vi "MuxReset.vi"(8 "error in (no error)":errorcluster, 11 "Pickering in":refnum<class "Pickering.lvclass">) -> (0 "error out":errorcluster, 3 "Pickering out":refnum<class "Pickering.lvclass">)   [LabVIEW 2013, in "Pickering.lvclass"]
uses:
  Pickering.lvclass
  PickeringMUX_CommandsGlobal.vi
  InstrControl.lvclass
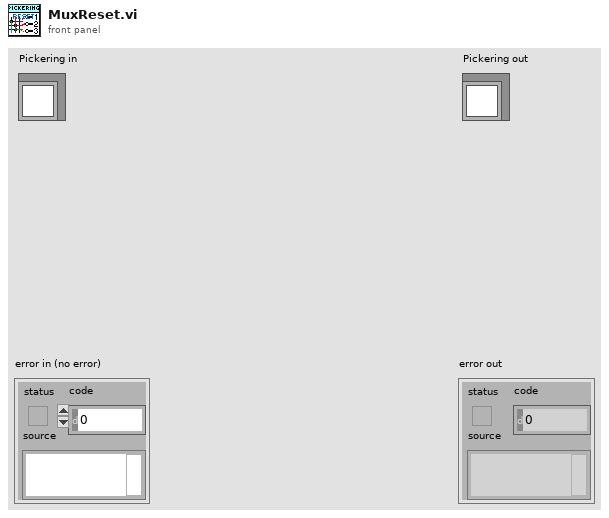
[diagram p1: front panel]
types:
  T1 = cluster{"Mux1 address":string, "Mux2 address":string, "Instrument name":string, "Instrument type":u16, "Command \"MUX Reset\"":string, "Command \"Select MUX Channel\"":string}
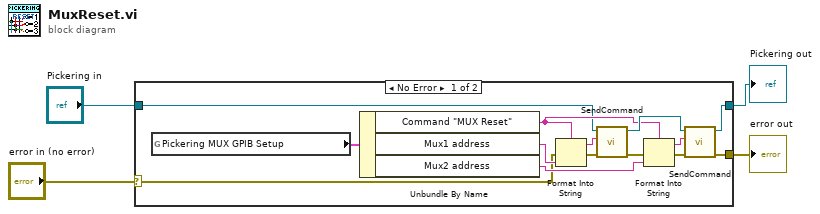
[diagram p0: block diagram]
diagram:
  n1 = case shown="No Error" "error in (no error)" {
    selector: "error in (no error)" -> [w6 w20]
    tunnel: [w13 w20] -> w4
    tunnel: [w17 w19] -> w3
    tunnel: "Pickering in" -> [w7 w19]
    frame No Error {
      n2 = global read "PickeringMUX_CommandsGlobal.vi" "Pickering MUX GPIB Setup"() -> (w5:T1)
      n3 = Unbundle By Name(w5) -> ("Command \"MUX Reset\""=w12:string, "Mux1 address"=w11:string, "Mux2 address"=w10:string)
      n4 = Format Into String(format string=w12, error in=w6, w11) -> (resulting string=w9:string, error out=w16:errorcluster)  [unwired: 1 in]
      n5 = call "SendCommand.vi"("error in (no error)"=w16, "Command string"=w9, "InstControl in"=w7) -> ("error out"=w15:errorcluster, "InstControl out"=w18:refnum<class "Pickering.lvclass">)  [unwired: 7 in]
      n6 = Format Into String(format string=w12, error in=w15, w10) -> (resulting string=w8:string, error out=w14:errorcluster)  [unwired: 1 in]
      n7 = call "SendCommand.vi"("error in (no error)"=w14, "Command string"=w8, "InstControl in"=w18) -> ("error out"=w13:errorcluster, "InstControl out"=w17:refnum<class "Pickering.lvclass">)  [unwired: 7 in]
    }
    frame Error {
    }
  }
  "error out" <- w4
  "Pickering out" <- w3
